vi "MergePeaks.vi"(10 "Array":dbl[][](array[numeric]), 11 "Smoothed Data":dbl[](array[numeric])) -> ()   [LabVIEW 2015]
uses:
  <userlib>/_OpenG.lib/array/array.llb/Remove Duplicates from 1D Array (DBL)__ogtk.vi
panel:
  out "Array 3":dbl[](array[numeric])
  out "Array 4":dbl[](array[numeric])
  out "Array 2":bool[](array[boolean])
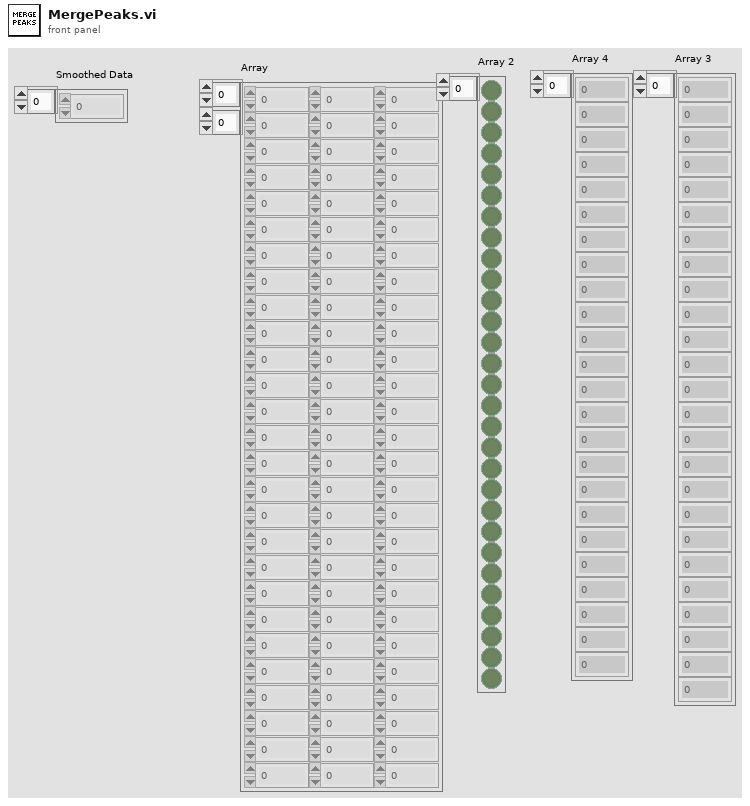
[diagram p1: front panel]
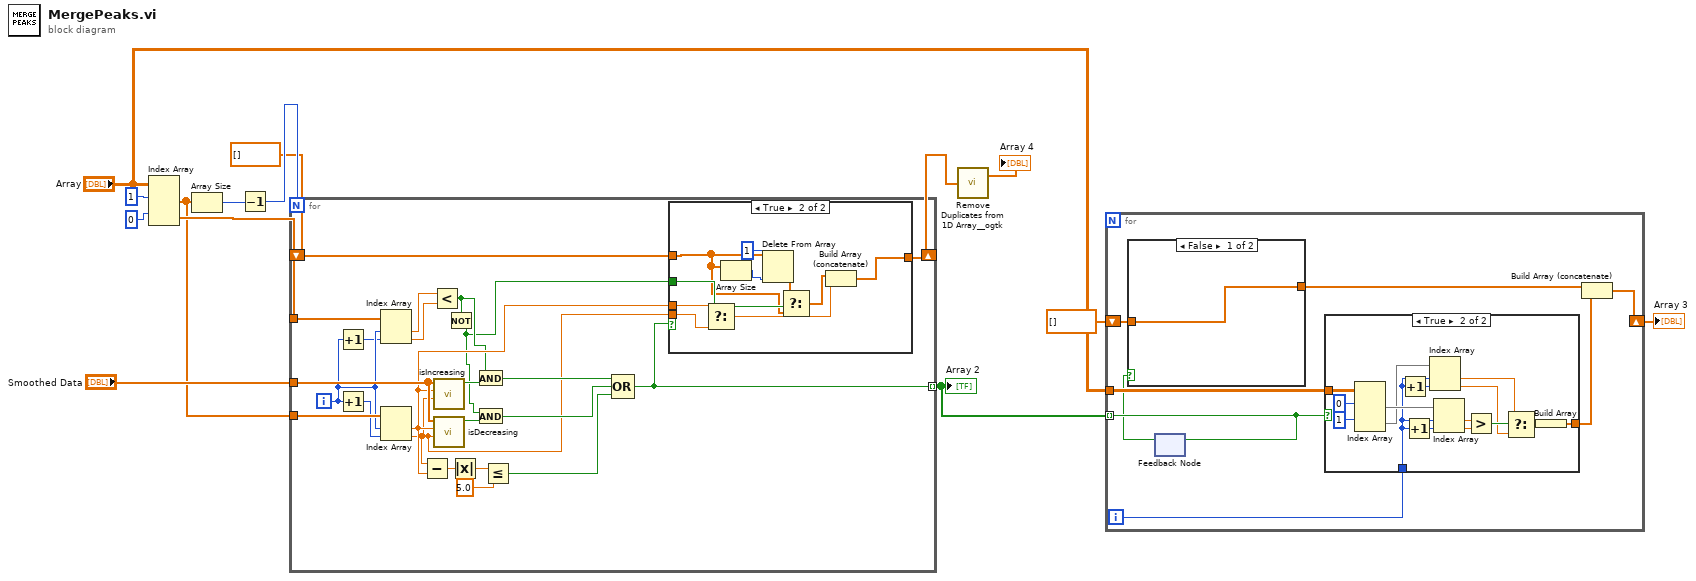
[diagram p0: block diagram]
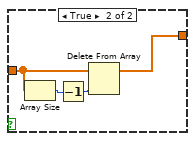
[diagram p2: hidden frame]
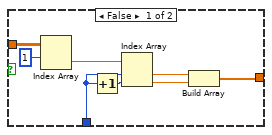
[diagram p3: hidden frame]
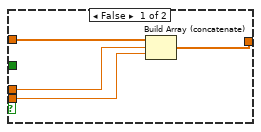
[diagram p4: hidden frame]
diagram:
  n1 = Index Array(array="Array", index (row) #1=1 ("index (row)"), index (row) #2=0 ("index (row)")) -> (element #1=w9:dbl[], element #2=w14:dbl[])  [unwired: 2 in]
  n2 = Array Size(array=w9) -> (size(s)=w10:i32)
  n3 = Decrement(x=w10) -> (x-1=w11:i32)
  n4 = for {
    N: w11 -> [_]
    tunnel: "Smoothed Data" -> [w34]
    tunnel: w9 -> [w37]
    tunnel: w14 -> [w31]
    tunnel: [w19] -> w4 mode=indexing
    shift-right: [w17] -> w6
    shift-left: dbl[] [] -> [w16]
    i -> [w30]
    n5 = Increment(x=w30) -> (x+1=w29:i32)
    n6 = Increment(x=w30) -> (x+1=w35:i32)
    n7 = Index Array(array=w31, index #1=w30, index #2=w29) -> (element #1=w23:dbl, element #2=w22:dbl)
    n8 = Index Array(array=w37, index #1=w30, index #2=w35) -> (element #1=w21:dbl, element #2=w20:dbl)
    n9 = Subtract(x=w20, y=w21) -> (x-y=w28:dbl)
    n10 = Less?(x=w23, y=w22) -> (x < y?=w18:bool)
    n11 = call "isIncreasing.vi"("End Index"=w20, "Start Index"=w21, "Array"=w34) -> ("isIncreasing?"=w36:bool)  [unwired: 8 in]
    n12 = call "isDecreasing.vi"("End Index"=w20, "Start Index"=w21, "Array"=w34) -> ("isDecreasing?"=w33:bool)  [unwired: 8 in]
    n13 = Not(x=w18) -> (.not. x?=w15:bool)
    n14 = Absolute Value(x=w28) -> (abs(x)=w27:dbl)
    n15 = And(x=w18, y=w36) -> (x .and. y?=w32:bool)
    n16 = And(x=w15, y=w33) -> (x .and. y?=w25:bool)
    n17 = Less Or Equal?(x=w27, y=5.0) -> (x <= y?=w24:bool)
    n18 = Compound Arithmetic op=OR(w32, w25, w24) -> (w19:bool)
    n19 = case shown="True" w19 {
      tunnel: w21 -> [w39 w51]
      tunnel: w20 -> [w38 w50]
      tunnel: [w40 w48] -> w17
      tunnel: w16 -> [w41 w43]
      tunnel: w15 -> [_ w45]
      frame False {
        n20 = Build Array (concatenate)(w41, w39, w38) -> (w40:dbl[])
      }
      frame True {
        n21 = Select(t=w51, s=w45, f=w50) -> (s? t:f=w49:dbl)
        n22 = Array Size(array=w43) -> (size(s)=w47:i32)
        n23 = Delete From Array(array=w43, length=1, index=w47) -> (array with subset deleted=w44:dbl[])  [unwired: 1 out]
        n24 = Select(t=w44, s=w45, f=w43) -> (s? t:f=w42:dbl[])
        n25 = Build Array (concatenate)(w42, w49) -> (w48:dbl[])
      }
    }
  }
  "Array 2" <- w4
  n26 = call-poly <userlib>:"Remove Duplicates from 1D Array__ogtk.vi"("Input Array"=w6) -> ("Output Array"=→"Array 4":dbl[])  [unwired: 1 out]
  n27 = for {
    tunnel: w4 -> [w57] mode=indexing
    tunnel: "Array" -> [w59]
    shift-right: [w52] -> w1
    shift-left: dbl[] [] -> [w55]
    i -> [w58]
    n28 = feedback-in #1(w57) -> ()
    n29 = feedback #1() -> (w56:bool)  [unwired: 1 in]
    n30 = case shown="False" w56 {
      tunnel: w55 -> [w60 w64]
      tunnel: [w60 w61] -> w54
      frame False {
      }
      frame True {
        n31 = Array Size(array=w64) -> (size(s)=w63:i32)
        n32 = Decrement(x=w63) -> (x-1=w62:i32)
        n33 = Delete From Array(array=w64, index=w62) -> (array with subset deleted=w61:dbl[])  [unwired: 1 in, 1 out]
      }
    }
    n34 = case shown="True" w57 {
      tunnel: w59 -> [w72 w87]
      tunnel: w58 -> [w69 w75]
      tunnel: [w65 w79] -> w53
      frame False {
        n35 = Index Array(array=w72, index (row)=1) -> (element=w70:dbl[])  [unwired: 1 in]
        n36 = Increment(x=w69) -> (x+1=w68:i32)
        n37 = Index Array(array=w70, index #1=w69, index #2=w68) -> (element #1=w67:dbl, element #2=w66:dbl)
        n38 = Build Array(w67, w66) -> (w65:dbl[])
      }
      frame True {
        n39 = Index Array(array=w87, index (row) #1=0 ("index (row)"), index (row) #2=1 ("index (row)")) -> (element #1=w85:dbl[], element #2=w76:dbl[])  [unwired: 2 in]
        n40 = Increment(x=w75) -> (x+1=w77:i32)
        n41 = Increment(x=w75) -> (x+1=w84:i32)
        n42 = Index Array(array=w76, index #1=w75, index #2=w77) -> (element #1=w74:dbl, element #2=w73:dbl)
        n43 = Index Array(array=w85, index #1=w75, index #2=w84) -> (element #1=w82:dbl, element #2=w81:dbl)
        n44 = Greater?(x=w82, y=w81) -> (0:w83:bool)
        n45 = Select(t=w74, s=w83, f=w73) -> (s? t:f=w80:dbl)
        n46 = Build Array(w80) -> (w79:dbl[])
      }
    }
    n47 = Build Array (concatenate)(w54, w53) -> (w52:dbl[])
  }
  "Array 3" <- w1
